vi "Station Search For Class Paths.vi"(0 "VI select":string(combo)="_Intialize.vi", 5 "Instrument Info":string[][](array[string]), 11 "error in (no error)":errorcluster) -> (4 "Updated Inst Info":string[][](array[string]), 15 "error out":errorcluster)   [LabVIEW 2018, in "Station.lvclass"]
uses:
  Station.lvclass
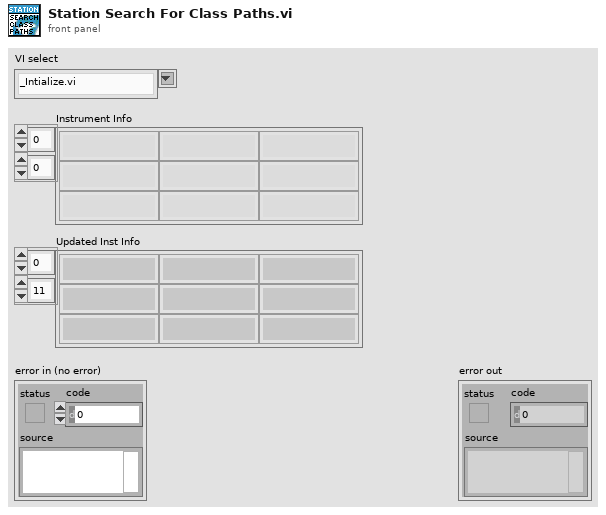
[diagram p1: front panel]
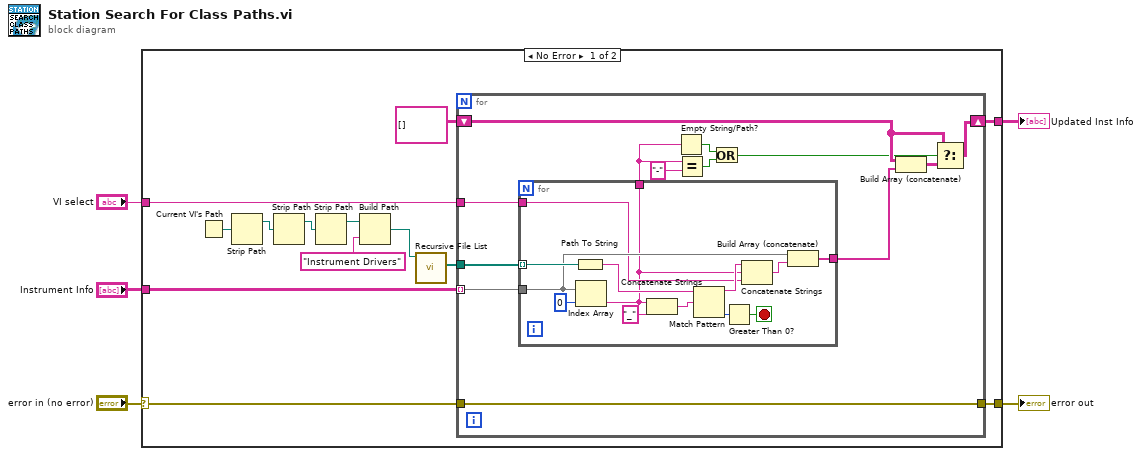
[diagram p0: block diagram]
diagram:
  n1 = case shown="No Error" "error in (no error)" {
    selector: "error in (no error)" -> [w18 w45]
    tunnel: [w17 w45] -> w1
    tunnel: "VI select" -> [w15 _]
    tunnel: "Instrument Info" -> [w14 _]
    tunnel: [w13 _] -> w3
    frame No Error {
      n2 = Current VI's Path() -> (path=w11:path)
      n3 = Strip Path(path=w11) -> (stripped path=w7:path)  [unwired: 1 out]
      n4 = Strip Path(path=w7) -> (stripped path=w6:path)  [unwired: 1 out]
      n5 = Strip Path(path=w6) -> (stripped path=w8:path)  [unwired: 1 out]
      n6 = Build Path(base path=w8, name or relative path="Instrument Drivers") -> (appended path=w9:path)
      n7 = call <vilib>:"Recursive File List.vi"("Folder Path"=w9) -> ("All Files in Dir"=w16:path[])  [unwired: 6 in, 4 out]
      n8 = for {
        tunnel: w18 -> [w31]
        tunnel: [w31] -> w17
        tunnel: w14 -> [w30] mode=indexing
        tunnel: w16 -> [w28]
        tunnel: w15 -> [w29]
        shift-right: [w27] -> w13
        shift-left: string[][] [] -> [w24]
        n9 = for {
          tunnel: w28 -> [w41] mode=indexing
          tunnel: w30 -> [w39]
          tunnel: [w38] -> w26
          tunnel: w29 -> [w35]
          tunnel: [w32] -> w23
          stop <- w40 stop-if-true
          n10 = Path To String(path=w41) -> (string=w44:string)
          n11 = Index Array(array=w39, index=0) -> (element=w32:string)
          n12 = Concatenate Strings(w32, "_" ("string")) -> (w34:string)
          n13 = Match Pattern(string=w44, regular expression=w34) -> (before substring=w36:string, offset past match=w43:i32)  [unwired: 1 in, 2 out]
          n14 = Greater Than 0?(x=w43) -> (x > 0?=w40:bool)
          n15 = Concatenate Strings(w36, w32, w35) -> (w37:string)
          n16 = Build Array (concatenate)(w39, w37) -> (w38:string[])
        }
        n17 = Empty String/Path?(string/path=w23) -> (empty?=w21:bool)
        n18 = Equal?(x=w23, y="-") -> (x = y?=w20:bool)
        n19 = Or(x=w21, y=w20) -> (x .or. y?=w19:bool)
        n20 = Build Array (concatenate)(w24, w26) -> (w25:string[][])
        n21 = Select(t=w24, s=w19, f=w25) -> (s? t:f=w27:string[][])
      }
    }
    frame Error {
    }
  }
  "error out" <- w1
  "Updated Inst Info" <- w3
